vi "Write Report Name.vi"(8 "error in (no error)":errorcluster, 10 "Report Name":string, 11 "Report In":refnum<class "Test Report.lvclass">) -> (0 "error out":errorcluster, 3 "Report Out":refnum<class "Test Report.lvclass">)   [LabVIEW 2020, in "Test Report.lvclass"]
uses:
  Test Report.lvclass
  Test Report.lvclass/Test Report.ctl
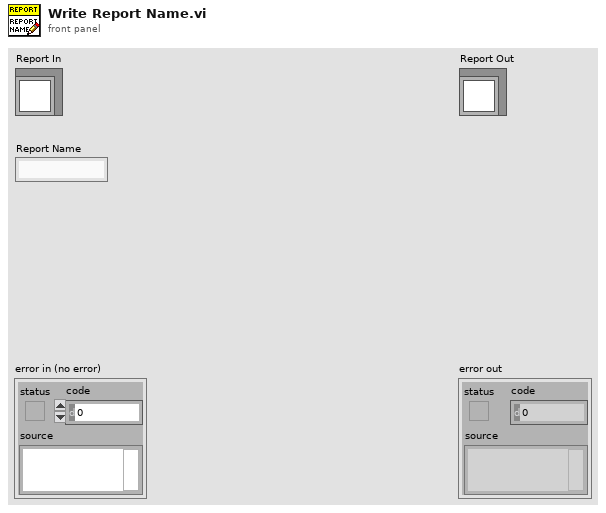
[diagram p1: front panel]
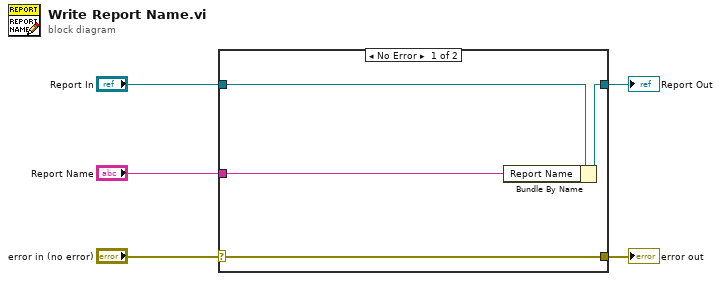
[diagram p0: block diagram]
diagram:
  n1 = case shown="No Error" "error in (no error)" {
    selector: "error in (no error)" -> [w9 w10]
    tunnel: [w9 w10] -> w4
    tunnel: [w7 w11] -> w2
    tunnel: "Report In" -> [w8 w11]
    tunnel: "Report Name" -> [w6 _]
    frame No Error {
      n2 = Bundle By Name(cluster=w8, "Report Name"=w6) -> (w7:refnum<class "Test Report.lvclass">)
    }
    frame Error {
    }
  }
  "error out" <- w4
  "Report Out" <- w2
